vi "Requester.vi"() -> ()   [LabVIEW 2024]
uses:
  src/NATS Client/NATS Client.lvclass/NATS Client.ctl
  src/NATS Subscription/NATS Subscription.lvclass
  src/NATS Client/NATS Client.lvclass
panel:
  out "Response Payload":string
  in  "Request Payload":string="please fix"
  out "error out":errorcluster
  out "loop error":errorcluster
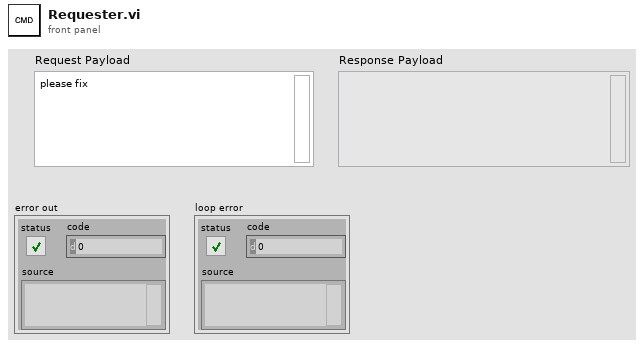
[diagram p1: front panel]
types:
  T1 = typedef "NATS Core.lvlib/nats message.ctl" = cluster{"subject":string, "payload":string, "sub id":string, "reply-to":string, "headers":string, "type":T2, "received":timestamp}
  T2 = typedef "NATS Core.lvlib/msg type.ctl" = enum16{"Undefined", "MSG", "HMSG", "+OK", "PING", "PONG", "-ERR", "INFO"}
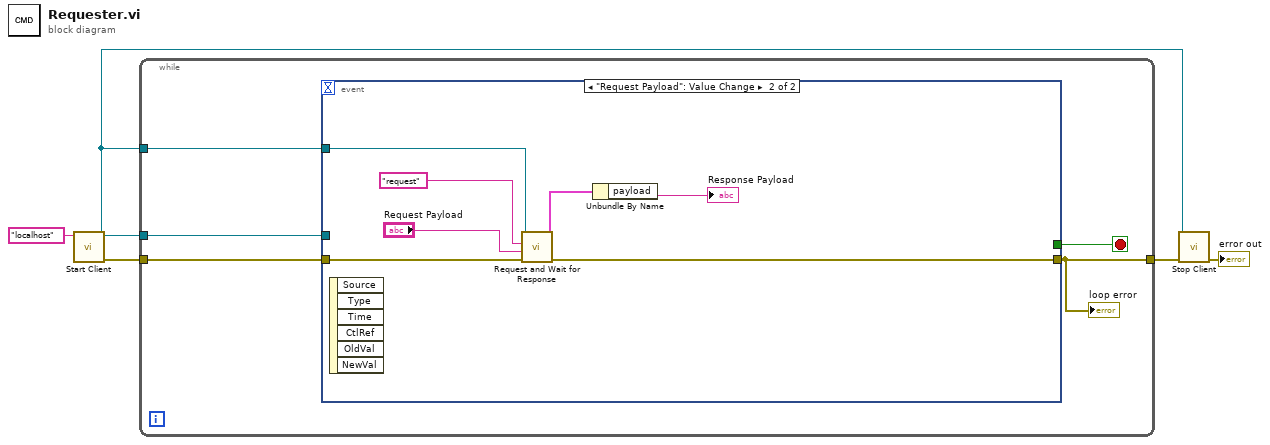
[diagram p0: block diagram]
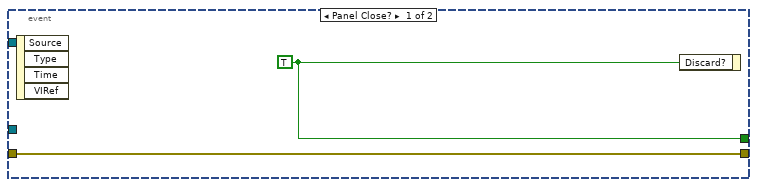
[diagram p2: hidden frame]
diagram:
  n1 = call "Start Client.vi"("address"="localhost") -> ("error out"=w5:errorcluster, "NATS Client out"=w2:refnum<class "NATS Client.lvclass">)  [unwired: 9 in]
  n2 = while {
    tunnel: w2 -> [w8]
    tunnel: w2 -> [w7]
    tunnel: w5 -> [w9]
    tunnel: [w6] -> w3
    stop <- w10 stop-if-true
    n3 = event shown="[1] \"Request Payload\": Value Change" {
      selector: _ -> [_ _]
      dyn-events: _ -> [_ _]
      timeout: _ -> [_ _]
      tunnel: [w12 _] -> w10
      tunnel: w9 -> [w11 w19]
      tunnel: [w11 w15] -> w6
      tunnel: w8 -> [_ _]
      tunnel: w7 -> [_ w18]
      event Panel Close? {
        w12 = TRUE ("Discard?")
        n4 = event-data() -> ()  [unwired: 1 in, 4 out]
        n5 = event-data("Discard?"=w12) -> ()  [unwired: 1 in, 1 out]
      }
      event "Request Payload": Value Change {
        n6 = event-data() -> ()  [unwired: 1 in, 6 out]
        n7 = call "Request and Wait for Response.vi"("error in"=w19, "payload"="Request Payload", "subject"="request" ("Subject"), "NATS Client in"=w18) -> ("error out"=w15:errorcluster, "nats message"=w14:T1)  [unwired: 5 in, 1 out]
        n8 = Unbundle By Name(w14) -> ("payload"=→"Response Payload":string)
      }
    }
    "loop error" <- w6
  }
  n9 = call "Stop Client.vi"("error in"=w3, "NATS Client"=w2) -> ("error out"=→"error out":errorcluster)  [unwired: 9 in]
